vi "Labspec MotorName2String.vi"(1 "Motor Name":T1) -> (0 "PositionName":string)   [LabVIEW 2014]
uses:
  MoveMotor Motor Name.ctl
panel:
  # "LICENSED MATERIALS – PROPERTY OF IBM\nCopyright IBM Corp. 2016,\nALL RIGHTS RESERVED"
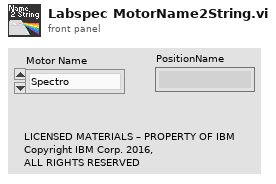
[diagram p1: front panel]
types:
  T1 = typedef "MoveMotor Motor Name.ctl" = enum16{"Spectro", "Premono", "Grating", "Slit", "Hole", "X", "Y", "XT", "YT", "XL", "YL", "Z", "Laser", "Filter", "Objective", "Detector", "Detector Temperature"}
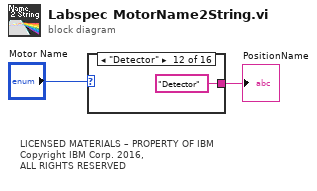
[diagram p0: block diagram]
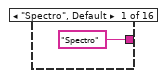
[diagram p2: hidden frame]
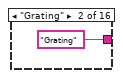
[diagram p3: hidden frame]
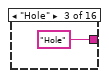
[diagram p4: hidden frame]
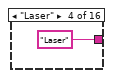
[diagram p5: hidden frame]
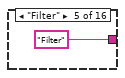
[diagram p6: hidden frame]
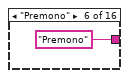
[diagram p7: hidden frame]
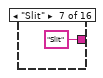
[diagram p8: hidden frame]
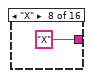
[diagram p9: hidden frame]
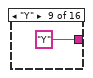
[diagram p10: hidden frame]
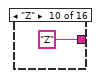
[diagram p11: hidden frame]
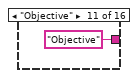
[diagram p12: hidden frame]
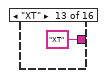
[diagram p13: hidden frame]
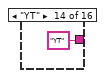
[diagram p14: hidden frame]
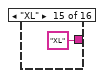
[diagram p15: hidden frame]
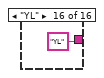
[diagram p16: hidden frame]
diagram:
  # "LICENSED MATERIALS – PROPERTY OF IBM\nCopyright IBM Corp. 2016,\nALL RIGHTS RESERVED"
  n1 = case shown="\"Detector\"" "Motor Name" {
    tunnel: ["Spectro" ("PositionName") "Grating" ("PositionName") "Hole" ("PositionName") "Laser" ("PositionName") "Filter" ("MotorName") "Premono" ("PositionName") "Slit" ("MotorName") "X" ("PositionName") "Y" ("PositionName") "Z" ("PositionName") "Objective" ("PositionName") "Detector" ("PositionName") "XT" ("PositionName") "YT" ("PositionName") "XL" ("PositionName") "YL" ("PositionName")] -> w1
    frame "Spectro", Default {
    }
    frame "Grating" {
    }
    frame "Hole" {
    }
    frame "Laser" {
    }
    frame "Filter" {
    }
    frame "Premono" {
    }
    frame "Slit" {
    }
    frame "X" {
    }
    frame "Y" {
    }
    frame "Z" {
    }
    frame "Objective" {
    }
    frame "Detector" {
    }
    frame "XT" {
    }
    frame "YT" {
    }
    frame "XL" {
    }
    frame "YL" {
    }
  }
  "PositionName" <- w1
